vi "Realsense Cam File Wrapper Create.vi"(6 "Identifier":string, 7 "Open? (T)":bool=TRUE, 8 "error in (no error)":errorcluster, 9 "Sensor Index (0)":i32, 10 "Device Index (0)":i32, 11 "Realsense Cam File Wrapper in":refnum<class "Realsense Cam File Wrapper.lvclass">) -> (0 "error out":errorcluster, 3 "Realsense Cam File Wrapper out":refnum<class "Realsense Cam File Wrapper.lvclass">)   [LabVIEW 2018, in "Realsense Cam File Wrapper.lvclass"]
uses:
  Realsense Cam File Wrapper.lvclass
  Realsense Cam File Wrapper.lvclass/Realsense Cam File Wrapper.ctl
  Realsense Cam/Realsense Cam.lvclass
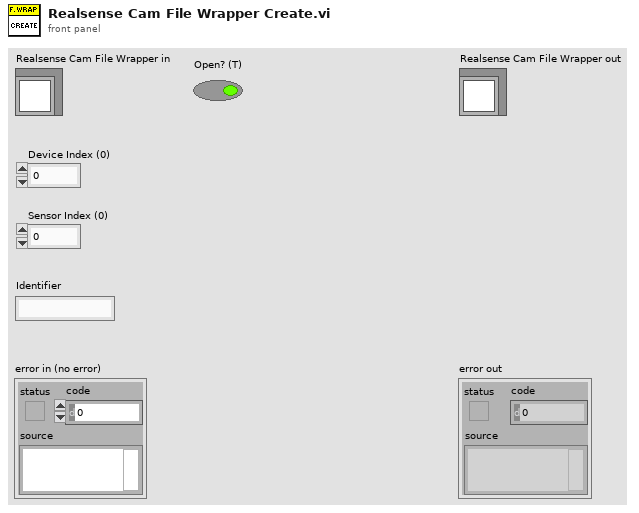
[diagram p1: front panel]
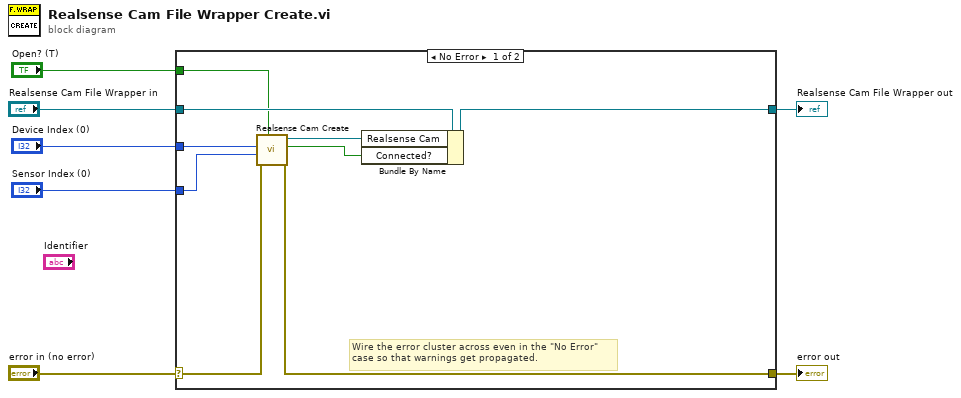
[diagram p0: block diagram]
diagram:
  n1 = case shown="No Error" "error in (no error)" {
    selector: "error in (no error)" -> [w9 w18]
    tunnel: [w8 w18] -> w6
    tunnel: [w13 w17] -> w4
    tunnel: "Realsense Cam File Wrapper in" -> [w14 w17]
    tunnel: "Device Index (0)" -> [w16 _]
    tunnel: "Sensor Index (0)" -> [w15 _]
    tunnel: "Open? (T)" -> [w10 _]
    frame No Error {
      # "Wire the error cluster across even in the \"No Error\"\ncase so that warnings get propagated."
      n2 = call "Realsense Cam Create.vi"("Connect? (T)"=w10, "error in (no error)"=w9, "Sensor Index (0)"=w15, "Device Index (0)"=w16) -> ("error out"=w8:errorcluster, "Found?"=w11:bool, "Realsense Cam out"=w12:refnum<class "Realsense Cam.lvclass">)  [unwired: 4 in, 1 out]
      n3 = Bundle By Name(cluster=w14, "Realsense Cam"=w12, "Connected?"=w11) -> (w13:refnum<class "Realsense Cam File Wrapper.lvclass">)
    }
    frame Error {
    }
  }
  "error out" <- w6
  "Realsense Cam File Wrapper out" <- w4
